vi "Init Tree.vi"(11 "Tree In":refnum<vi>) -> (3 "Tree Out":refnum<vi>)   [LabVIEW 2020, in "Tree Browser.lvlib"]
doc: "Setup a tree for browsing directories on disk. Inserts a top level root node, then child nodes for each available disk (C:\\, D:\\, etc)."
uses:
  Tree Browser.lvlib
  Types/UTF-8 String/UTF-8 String.lvclass/UTF-8 String.ctl
  Types/UTF-8 String/UTF-8 String.lvclass
  G-Unicode.lvlib
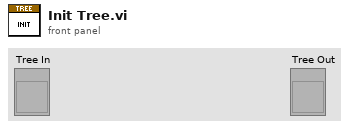
[diagram p1: front panel]
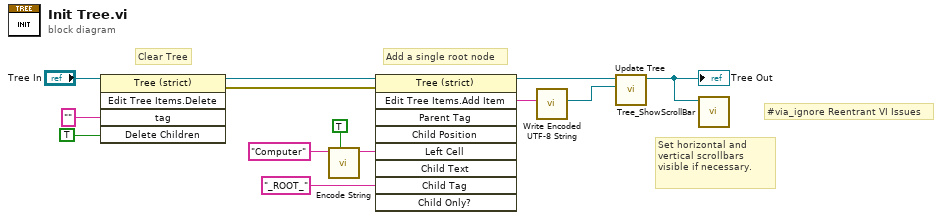
[diagram p0: block diagram]
diagram:
  # "#via_ignore Reentrant VI Issues"
  # "Set horizontal and vertical scrollbars visible if necessary."
  # "Add a single root node"
  # "Clear Tree"
  n1 = invoke class="Tree (strict)" method="Edit Tree Items.Delete"(reference="Tree In", "tag"="" ("Tag"), "Delete Children"=TRUE ("Delete Children?")) -> (reference out=w13:refnum<vi>, error out=w8:errorcluster)  [unwired: 2 in, 3 out]
  n2 = call "Encode String.vi"("Prepend BOM (F)"=TRUE, "String in"="Computer" ("Left Cell String")) -> ("String out"=w1:string)  [unwired: 8 in, 1 out]
  n3 = invoke class="Tree (strict)" method="Edit Tree Items.Add Item"(reference=w13, error in=w8, "Left Cell"=w1, "Child Tag"="_ROOT_") -> (reference out=w6:refnum<vi>, "Edit Tree Items:Add Item"=w7:string)  [unwired: 5 in, 7 out]
  n4 = call "Write Encoded UTF-8 String.vi"("Encoded UTF-8 String"=w7) -> ("UTF-8 String"=w4:refnum<class "UTF-8 String.lvclass">)  [unwired: 10 in]
  n5 = call "Update Tree.vi"("Parent Tag"=w4, "Tree In"=w6) -> ("Tree Out"=w5:refnum<vi>)  [unwired: 9 in]
  "Tree Out" <- w5
  n6 = call <vilib>:"Tree_ShowScrollBar.vi"("Tree"=w5) -> ()  [unwired: 10 in, 1 out]
